vi "_Read.vi"(8 "error in (no error)":errorcluster, 9 "Timeout S (0)":dbl, 10 "Bytes to Read (0)":i32, 11 "DeployTCPResource in":refnum<class "TCPResource.lvclass">) -> (0 "error out":errorcluster, 1 "Bytes Read":i32, 2 "Data":string, 3 "DeployTCPResource out":refnum<class "TCPResource.lvclass">)   [LabVIEW 2020, in "PicoG-Core.lvlib" / "TCPResource.lvclass"]
uses:
  TCPResource.lvclass
  TCPResource.lvclass/TCPResource.ctl
  <vilib>/IlluminatedG/lv-stream/stream/Stream.lvclass
  <vilib>/IlluminatedG/lv-stream-tcp/TCP Client/TCP Client.lvclass
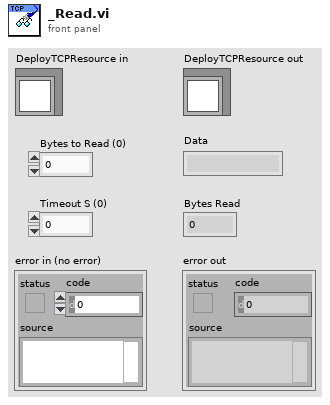
[diagram p1: front panel]
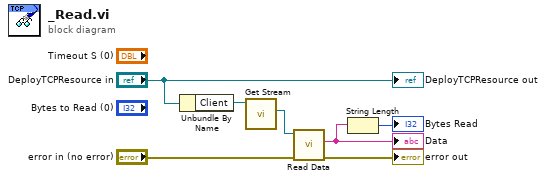
[diagram p0: block diagram]
diagram:
  n1 = Unbundle By Name("DeployTCPResource in") -> ("Client"=w7:refnum<class "TCP Client.lvclass">)
  n2 = call-dynamic "Get Stream.vi"("TCP Client in"=w7) -> ("Stream"=w6:refnum<class "Stream.lvclass">)  [unwired: 8 in, 2 out]
  n3 = call <vilib>:"Read Data.vi"("error in (no error)"="error in (no error)", "Stream in"=w6) -> ("error out"=→"error out":errorcluster, "Data"=w4:string)  [unwired: 7 in, 1 out]
  "Data" <- w4
  n4 = String Length(string=w4) -> (length=→"Bytes Read":i32)
  "DeployTCPResource out" <- "DeployTCPResource in"
